vi "DL-TCP Server.vi"(0 "callsign":string, 7 "TCP Event":refnum<user-event>) -> ()   [LabVIEW 2020]
uses:
  Typedefs/DL-Globals.vi
panel:
  out "error out":errorcluster
  out "Command":string
  out "Connected":bool
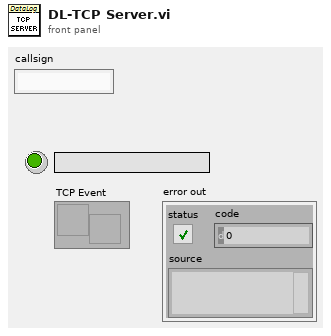
[diagram p1: front panel]
types:
  T1 = enum16{"big-endian, network order", "native, host order", "little-endian"}
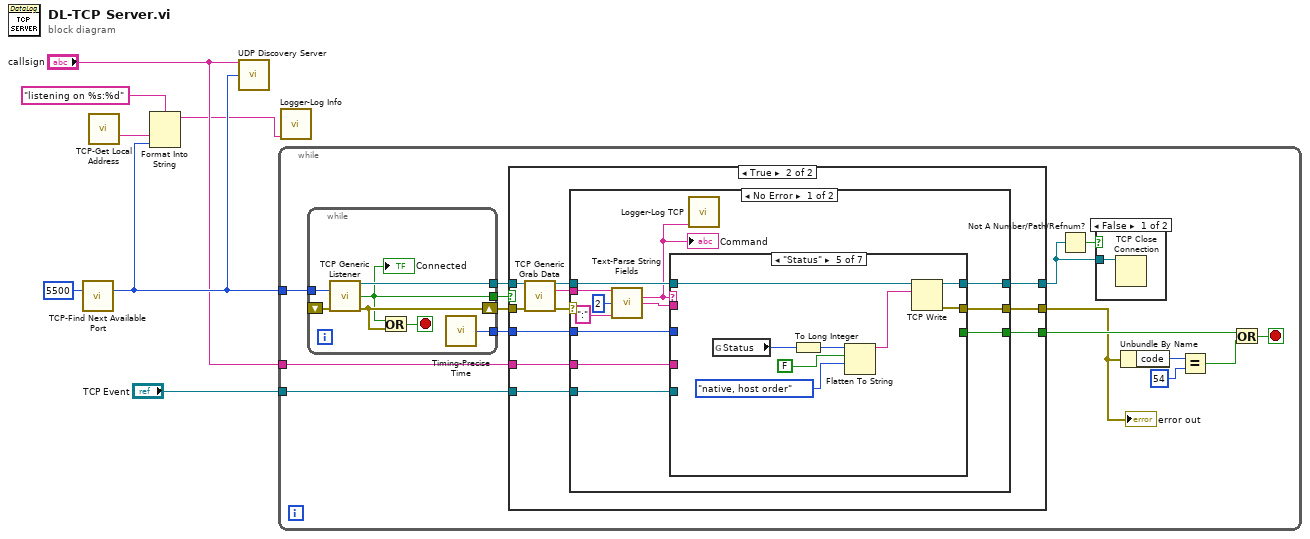
[diagram p0: block diagram]
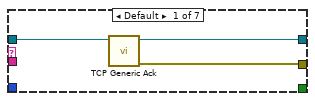
[diagram p3: hidden frame]
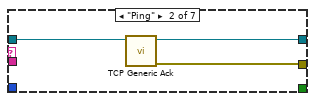
[diagram p4: hidden frame]
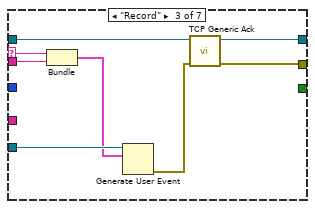
[diagram p5: hidden frame]
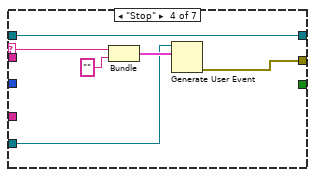
[diagram p6: hidden frame]
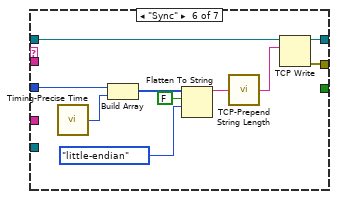
[diagram p7: hidden frame]
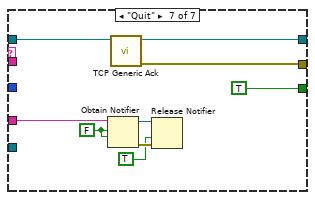
[diagram p8: hidden frame]
diagram:
  n1 = call "TCP-Find Next Available Port.vi"("start"=u16 5500) -> ("port"=w4:u16)  [unwired: 13 in, 1 out]
  n2 = call "TCP-Get Local Address.vi"() -> ("address"=w6:string)  [unwired: 14 in, 1 out]
  n3 = Format Into String(format string="listening on %s:%d" ("string"), w6, w4) -> (resulting string=w2:string)  [unwired: 2 in, 1 out]
  n4 = call "UDP Discovery Server.vi"("Name"="callsign", "Port"=w4) -> ()  [unwired: 13 in, 1 out]
  n5 = while {
    tunnel: w4 -> [w22]
    tunnel: "callsign" -> [w11]
    tunnel: "TCP Event" -> [w10]
    stop <- w13 stop-if-true
    n6 = while {
      tunnel: w22 -> [w29]
      shift-right: [w26] -> w21
      shift-left: _ -> [w28]
      tunnel: [w24] -> w20
      tunnel: [w27] -> w19
      tunnel: [w23] -> w9
      stop <- w25 stop-if-true
      n7 = call "TCP Generic Listener.vi"("port"=w29, "error in (no error)"=w28) -> ("connection ID"=w27:refnum<k5>, "Connected?"=w24:bool, "error out"=w26:errorcluster)  [unwired: 11 in]
      "Connected" <- w24
      n8 = Or(x=w24, y=w26) -> (x .or. y?=w25:bool)
      n9 = call "Timing-Precise Time.vi"() -> ("preciseTime"=w23:i64)  [unwired: 15 in]
    }
    n10 = case shown="True" w20 {
      tunnel: w21 -> [w30 w41]
      tunnel: w19 -> [w31 w42]
      tunnel: [w31 w34] -> w17
      tunnel: [w30 w33] -> w8
      tunnel: [_ w37] -> w16
      tunnel: w11 -> [_ w36]
      tunnel: w10 -> [_ w35]
      tunnel: w9 -> [_ w32]
      frame False {
      }
      frame True {
        n11 = call "TCP Generic Grab Data.vi"("connection ID"=w42, "error in (no error)"=w41) -> ("connection ID out"=w38:refnum<k5>, "data out"=w40:string, "error out"=w39:errorcluster)  [unwired: 11 in]
        n12 = case shown="No Error" w39 {
          selector: w39 -> [_ w102]
          tunnel: w40 -> [w48 _]
          tunnel: w38 -> [w54 w103]
          tunnel: [w53 w103] -> w34
          tunnel: [w52 w102] -> w33
          tunnel: [w51 _] -> w37
          tunnel: w36 -> [w50 _]
          tunnel: w35 -> [w49 _]
          tunnel: w32 -> [w43 _]
          frame No Error {
            n13 = call "Text-Parse String Fields.vi"("String"=w48, "Max fields"=2, "Separator"=":") -> ("element"=w47:string, "element 2"=w46:string)  [unwired: 7 in, 4 out]
            "Command" <- w47
            n14 = case shown="\"Status\"" w47 {
              selector: w47 -> [_ _ w67 w72 _ _ _]
              tunnel: w54 -> [w57 w60 w64 w74 w80 w89 w95]
              tunnel: [w56 w59 w61 w74 w82 w90 w94] -> w53
              tunnel: [w55 w58 w62 w73 w81 w88 w93] -> w52
              tunnel: [_ _ _ _ _ _ TRUE] -> w51
              tunnel: w46 -> [_ _ w66 _ _ _ _]
              tunnel: w50 -> [_ _ _ _ _ _ w96]
              tunnel: w49 -> [_ _ w68 w69 _ _ _]
              tunnel: w43 -> [_ _ _ _ _ w92 _]
              frame Default {
                n15 = call "TCP Generic Ack.vi"("connection ID"=w57) -> ("error out"=w55:errorcluster, "connection ID out"=w56:refnum<k5>)  [unwired: 9 in]
              }
              frame "Ping" {
                n16 = call "TCP Generic Ack.vi"("connection ID"=w60) -> ("error out"=w58:errorcluster, "connection ID out"=w59:refnum<k5>)  [unwired: 9 in]
              }
              frame "Record" {
                n17 = Bundle(w67, "element 2"=w66) -> (w65:cluster{string, "element 2":string})  [unwired: 1 in]
                n18 = Generate User Event(user event=w68, event data cluster=w65) -> (error out=w63:errorcluster)  [unwired: 2 in, 1 out]
                n19 = call "TCP Generic Ack.vi"("error in (no error)"=w63, "connection ID"=w64) -> ("error out"=w62:errorcluster, "connection ID out"=w61:refnum<k5>)  [unwired: 8 in]
              }
              frame "Stop" {
                n20 = Bundle(w72, "") -> (w70:cluster{string, string})  [unwired: 1 in]
                n21 = Generate User Event(user event=w69, event data cluster=w70) -> (error out=w73:errorcluster)  [unwired: 2 in, 1 out]
              }
              frame "Status" {
                n22 = global read "DL-Globals.vi" "Status"() -> (w75:enum16{"Idle", "Record", "Error"})
                n23 = To Long Integer(number=w75) -> (32bit integer=w76:i32)
                n24 = Flatten To String(anything=w76, prepend array or string size? (T)=FALSE, byte order (0:big-endian, network order)=T1."native, host order") -> (data string=w78:string)  [unwired: 1 in, 2 out]
                n25 = TCP Write(connection ID=w80, data in=w78) -> (connection ID out=w82:refnum<k5>, error out=w81:errorcluster)  [unwired: 2 in, 1 out]
              }
              frame "Sync" {
                n26 = call "Timing-Precise Time.vi"() -> ("preciseTime"=w91:i64)  [unwired: 15 in]
                n27 = Build Array(w92, w91) -> (w87:i64[])
                n28 = Flatten To String(anything=w87, prepend array or string size? (T)=FALSE, byte order (0:big-endian, network order)=T1."little-endian") -> (data string=w84:string)  [unwired: 1 in, 2 out]
                n29 = call "TCP-Prepend String Length.vi"("Command"=w84) -> ("String"=w83:string)  [unwired: 4 in]
                n30 = TCP Write(connection ID=w89, data in=w83) -> (connection ID out=w90:refnum<k5>, error out=w88:errorcluster)  [unwired: 2 in, 1 out]
              }
              frame "Quit" {
                w97 = FALSE
                n31 = Obtain Notifier(name (unnamed)=w96, notification data type=w97, create if not found? (T)=w97) -> (notifier out=w100:refnum<notifier>, error out=w99:errorcluster)  [unwired: 1 in, 1 out]
                n32 = call "TCP Generic Ack.vi"("connection ID"=w95) -> ("error out"=w93:errorcluster, "connection ID out"=w94:refnum<k5>)  [unwired: 9 in]
                n33 = Release Notifier(notifier=w100, force destroy? (F)=TRUE, error in (no error)=w99) -> ()  [unwired: 3 out]
              }
            }
            n34 = call "Logger-Log TCP.vi"("Message"=w47) -> ()  [unwired: 14 in, 1 out]
          }
          frame Error {
          }
        }
      }
    }
    "error out" <- w8
    n35 = Not A Number/Path/Refnum?(number/path/refnum=w17) -> (NaN/Path/Refnum?=w18:bool)
    n36 = case shown="False" w18 {
      tunnel: w17 -> [w104 _]
      frame False {
        n37 = TCP Close Connection(connection ID=w104) -> ()  [unwired: 2 in, 2 out]
      }
      frame True {
      }
    }
    n38 = Unbundle By Name(w8) -> ("code"=w15:i32)
    n39 = Equal?(x=w15, y=54) -> (x = y?=w12:bool)
    n40 = Or(x=w16, y=w12) -> (x .or. y?=w13:bool)
  }
  n41 = call "Logger-Log Info.vi"("Message"=w2) -> ()  [unwired: 14 in, 1 out]
